vi "Subvi pulse stretcher.vi"(9 "Input":bool) -> (1 "Output":bool)   [LabVIEW 2017]
uses:
  GV stage pulse stretcher.vi
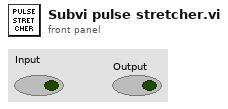
[diagram p1: front panel]
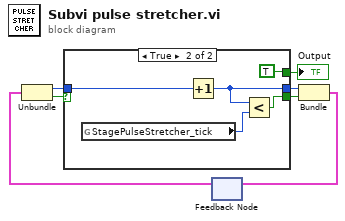
[diagram p0: block diagram]
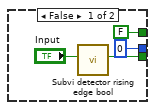
[diagram p2: hidden frame]
diagram:
  n1 = feedback #1() -> (w3:cluster{u32, "Output":bool})  [unwired: 1 in]
  n2 = Unbundle(w3) -> (w6:u32, "Output"=w7:bool)
  n3 = case shown="True" w7 {
    tunnel: [FALSE TRUE] -> w1
    tunnel: [w9 w15] -> w4
    tunnel: [u32 0 w14] -> w5
    tunnel: w6 -> [_ w13]
    frame False {
      n4 = call "Subvi detector rising edge bool.vi"("Input"="Input") -> ("Output"=w9:bool)  [unwired: 10 in]
    }
    frame True {
      n5 = global read "GV stage pulse stretcher.vi" "StagePulseStretcher_tick"() -> (w12:u32)
      n6 = Increment(x=w13) -> (x+1=w14:u32)
      n7 = Less?(x=w14, y=w12) -> (x < y?=w15:bool)
    }
  }
  "Output" <- w1
  n8 = Bundle(w5, "Output"=w4) -> (w2:cluster{u32, "Output":bool})  [unwired: 1 in]
  n9 = feedback-in #1(w2) -> ()
